vi "Read ADC.vi"(8 "error in (no error)":errorcluster, 9 "Canal":dbl, 10 "VISA resource name":refnum<visa-resource-name>, 11 "Arduino in":refnum<class "Arduino.lvclass">) -> (0 "error out":errorcluster, 1 "Response":string, 2 "VISA resource name 2":refnum<visa-resource-name>, 3 "Arduino out":refnum<class "Arduino.lvclass">)   [LabVIEW 2020, in "Arduino.lvclass"]
uses:
  Arduino.lvclass
  Abstract/Serial Device/Serial Device.lvclass
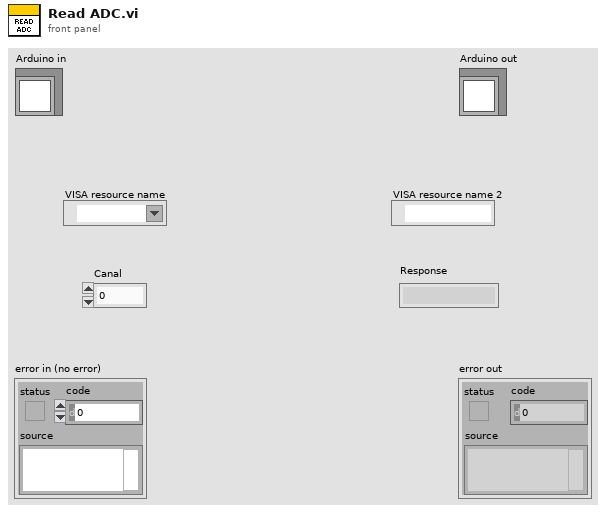
[diagram p1: front panel]
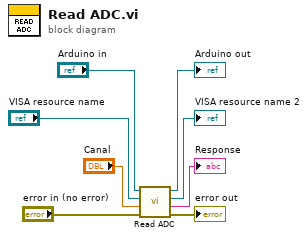
[diagram p0: block diagram]
diagram:
  n1 = call-parent "Read ADC.vi"("error in (no error)"="error in (no error)", "Canal"="Canal", "VISA resource name"="VISA resource name", "Serial Device in"="Arduino in") -> ("error out"=→"error out":errorcluster, "Response"=→"Response":string, "VISA resource name 2"=→"VISA resource name 2":refnum<visa-resource-name>, "Serial Device out"=→"Arduino out":refnum<class "Arduino.lvclass">)  [unwired: 4 in]
